vi "Open WorkSheet.vi"(2 "error in (no error)":errorcluster caption="错误输入（无错误）", 4 "Excel._Workbook":refnum<k7>) -> (0 "error out":errorcluster caption="错误输出", 1 "Excel._Worksheet":refnum<k7>)   [LabVIEW 2017]
doc: "按名称打开工作表。将应用程序引用句柄作为输入。如尚未连接名称或者字符串长度为零，将打开第一个工作表。"
panel:
  in  "Excel._Worksheet":refnum<k7>
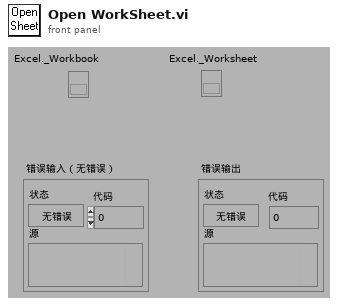
[diagram p1: front panel]
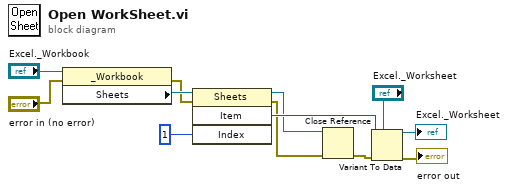
[diagram p0: block diagram]
diagram:
  n1 = property class="_Workbook"(reference="Excel._Workbook", error in="error in (no error)") -> (error out=w9:errorcluster, "Sheets"=w10:refnum<k7>)  [unwired: 1 out]
  n2 = invoke class="Sheets" method="Item"(reference=w10, error in=w9, "Index"=1) -> (reference out=w4:refnum<k7>, error out=w3:errorcluster, "Item"=w8:variant)  [unwired: 1 in, 1 out]
  n3 = Close Reference(reference=w4, error in (no error)=w3) -> (error out=w2:errorcluster)
  n4 = Variant To Data(error in=w2, type="Excel._Worksheet", Variant=w8) -> (data=→"Excel._Worksheet":refnum<k7>, error out=→"error out":errorcluster)
